vi "trial tdms.vi"() -> ()   [LabVIEW 2025]
uses:
  <vilib>/Platform/TimedLoop/XDataNode/timing_clust.ctl
  <vilib>/Platform/TimedLoop/XDataNode/nitl_modes.ctl
  <vilib>/Platform/TimedLoop/XDataNode/wakeup.ctl
  <vilib>/platform/TimedLoop/XDataNode/XDataNode.xnode
  <vilib>/Platform/TimedLoop/XDataNode/XDNodeRunTimeDep.lvlib
panel:
  in  "Stop":bool
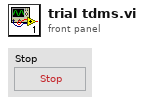
[diagram p1: front panel]
types:
  T1 = enum16{"open", "open or create", "create or replace", "create", "open (read-only)"}
  T2 = typedef "XDNodeRunTimeDep.lvlib/timing_clust.ctl" = cluster{"Expected End [f-1]":u64, "Actual End [f-1]":u64, "Finished Late? [f-1]":bool, "Expected End [i-1]":u64, "Actual End [i-1]":u64, "Finished Late? [i-1]":bool, "Expected Start [i]":u64, "Actual Start [i]":u64, "Expected Start [f]":u64, "Actual Start [f]":u64, "Source Name":string, "Structure Name":string, "Period":i64, "Deadline":i64, "Offset":i64, "Start":i64, "Priority":i32, "Timeout":i32, "Mode":T3, "Wakeup Reason":T4, "Error":errorcluster, "Source Type":string, "Secondary Source Type":string, "Global End Time":u64, "Global Start Time":u64, "Frame Duration":u64, "Iteration Duration":u64, "Assigned CPU":i32, "I/O Scan Engine Mode":u32}
  T3 = typedef "XDNodeRunTimeDep.lvlib/nitl_modes.ctl" = enum32{"No Change", "Process missed periods, maintain original phase", "Discard missed periods, maintain original phase", "Process missed periods, ignore original phase", "Discard missed periods, ignore original phase"}
  T4 = typedef "XDNodeRunTimeDep.lvlib/wakeup.ctl" = enum32{"Normal", "Aborted", "Asynchronous wakeup", "Timing source error", "Timed loop error", "Timeout"}
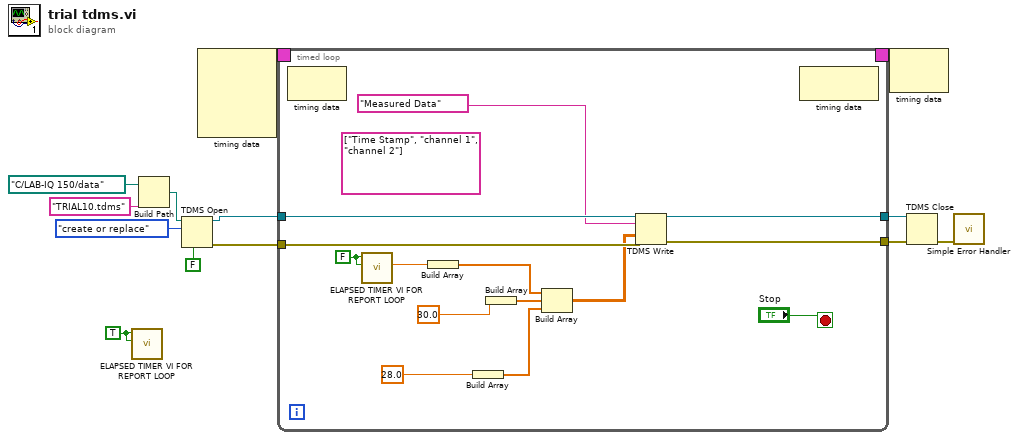
[diagram p0: block diagram]
diagram:
  w1 = TRUE ("PAUSE")
  n1 = call "ELAPSED TIMER VI FOR REPORT LOOP.vi"("RESET"=w1, "PAUSE"=w1) -> ()  [unwired: 7 in, 3 out]
  n2 = Build Path(base path=path "C:/LAB-IQ 150/data", name or relative path="TRIAL10.tdms") -> (appended path=w12:path)
  n3 = TDMS Open(6:FALSE ("disable buffering (T)"), 10:T1."create or replace" ("operation"), 11:w12) -> (0:w8:errorcluster, 3:w7:refnum<k34>)  [unwired: 4 in]
  n4 = node-c288() -> (w3:T2)  [unwired: 4 in]
  n5 = timed-loop {
    tunnel: w8 -> [w27]
    tunnel: w7 -> [w26]
    tunnel: [w25] -> w5
    tunnel: [w24] -> w4
    timing: w3 -> [_]
    timing-out: [_] -> w2
    stop <- "Stop" stop-if-true
    (unwired) string[] ["Time Stamp", "channel 1", "channel 2"] ("channel name(s) in (Untitled)")
    w22 = FALSE ("PAUSE")
    n6 = node-c288() -> ()  [unwired: 1 in, 1 out]
    n7 = call "ELAPSED TIMER VI FOR REPORT LOOP.vi"("RESET"=w22, "PAUSE"=w22) -> ("ELAPSED TIMER"=w21:dbl)  [unwired: 7 in, 2 out]
    n8 = Build Array(w21) -> (w16:dbl[])
    n9 = Build Array(28.0 ("element")) -> (w14:dbl[])
    n10 = Build Array(30.0 ("element")) -> (w15:dbl[])
    n11 = Build Array(w16, w15, w14) -> (w20:dbl[][])
    n12 = TDMS Write(0:w26, 5:"Measured Data" ("group name"), 9:w20, 11:w27) -> (4:w24:refnum<k34>, 15:w25:errorcluster)  [unwired: 2 in, 2 out]
    n13 = node-c288() -> ()  [unwired: 1 in, 1 out]
  }
  n14 = node-c288(w2) -> ()  [unwired: 1 out]
  n15 = TDMS Close(8:w5, 11:w4) -> (0:w6:errorcluster)  [unwired: 1 out]
  n16 = call <vilib>:"Simple Error Handler.vi"("error in (no error)"=w6) -> ()  [unwired: 2 in, 7 out]
